vi "Excel_Update_Chart.vi"(0 "Excel._Worksheet":refnum<k7>, 1 "chart data":dbl[][](array[numeric]) format="%0.2f", 5 "Shapes":refnum<k7>, 9 "Chart index":u16, 11 "error in (no error)":errorcluster, 12 "column header":string[](array[string]), 13 "row header":string[](array[string])) -> (15 "error out":errorcluster)   [LabVIEW 2020, in "NI_ReportGenerationToolkit.lvlib"]
uses:
  <vilib>/addons/_office/NI_ReportGenerationToolkit.lvlib
panel:
  in  "MS Graph":refnum<k7>
  in  "Excel._OLEObject":refnum<k7>
  in  "Graph.Chart":refnum<k7>
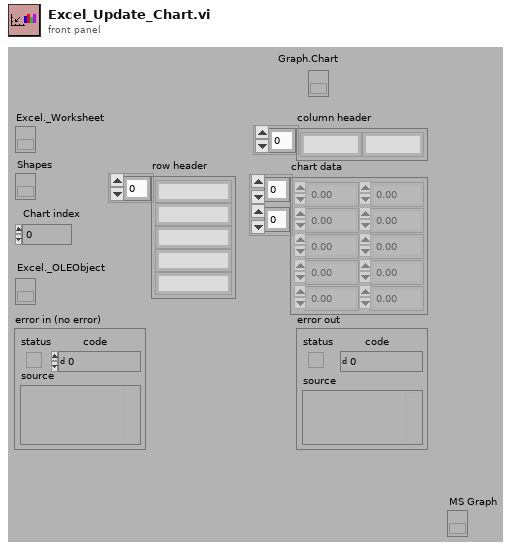
[diagram p1: front panel]
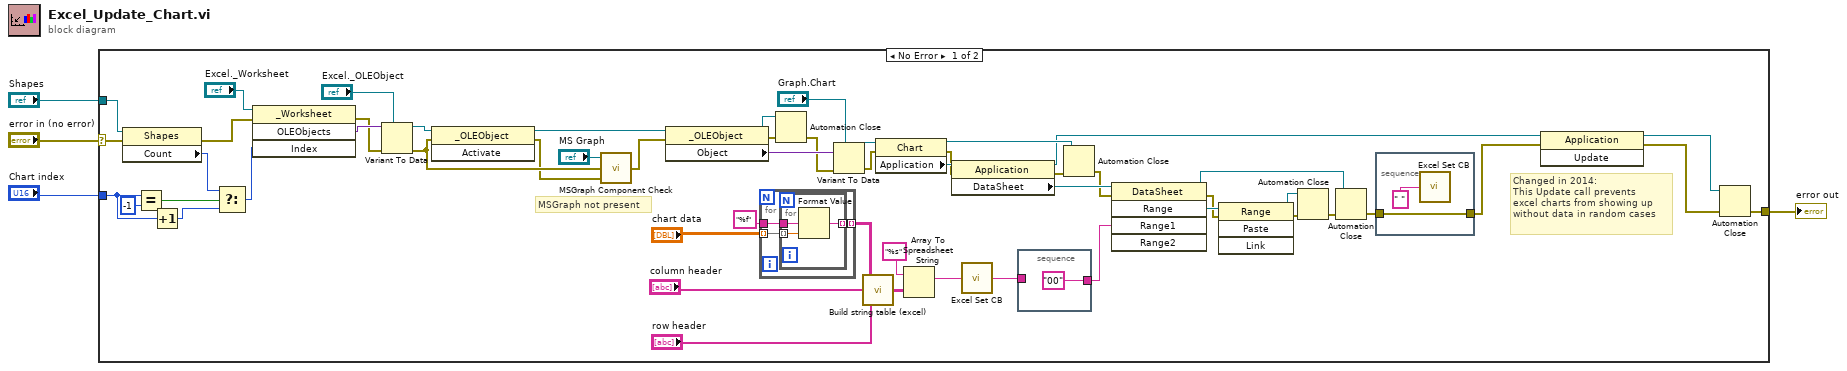
[diagram p0: block diagram]
diagram:
  n1 = case shown="No Error" "error in (no error)" {
    selector: "error in (no error)" -> [w9 w68]
    tunnel: "Chart index" -> [w46 _]
    tunnel: [w19 w68] -> w3
    tunnel: "Shapes" -> [w17 _]
    frame No Error {
      # "Changed in 2014:\nThis Update call prevents\nexcel charts from showing up \nwithout data in random cases"
      # "MSGraph not present"
      n2 = property class="Shapes"(reference=w17, error in=w9) -> (error out=w49:errorcluster, "Count"=w48:i32)  [unwired: 1 out]
      n3 = Equal?(x=w46, y=i16 -1) -> (x = y?=w57:bool)
      n4 = Increment(x=w46) -> (x+1=w55:u16)
      n5 = Select(t=w48, s=w57, f=w55) -> (s? t:f=w47:i32)
      n6 = invoke class="_Worksheet" method="OLEObjects"(reference="Excel._Worksheet", error in=w49, "Index"=w47) -> (error out=w52:errorcluster, "OLEObjects"=w53:variant)  [unwired: 1 in, 2 out]
      n7 = Variant To Data(error in=w52, type="Excel._OLEObject", Variant=w53) -> (data=w25:refnum<k7>, error out=w12:errorcluster)
      n8 = invoke class="_OLEObject" method="Activate"(reference=w25, error in=w12) -> (reference out=w24:refnum<k7>, error out=w11:errorcluster)  [unwired: 1 in, 1 out]
      n9 = call <vilib>:"MSGraph Component Check.vi"("error 2"=w11, "error 1"=w12, "MS Graph"="MS Graph") -> ("error out"=w10:errorcluster)
      n10 = property class="_OLEObject"(reference=w24, error in=w10) -> (reference out=w50:refnum<k7>, error out=w51:errorcluster, "Object"=w45:variant)
      n11 = for {
        tunnel: "chart data" -> [w64] mode=indexing
        tunnel: "%f" -> [w63]
        tunnel: [w62] -> w42 mode=indexing
        n12 = for {
          tunnel: w64 -> [w67] mode=indexing
          tunnel: w63 -> [w66]
          tunnel: [w65] -> w62 mode=indexing
          n13 = Format Value(format string=w66, value (0)=w67) -> (output string=w65:string)  [unwired: 1 out]
        }
      }
      n14 = Automation Close(3:w51, 5:w50) -> (0:w44:errorcluster)
      n15 = Variant To Data(error in=w44, type="Graph.Chart", Variant=w45) -> (data=w16:refnum<k7>, error out=w43:errorcluster)
      n16 = call <vilib>:"Build string table (excel).vi"("row headers"="row header", "column headers"="column header", "text data"=w42) -> ("output table"=w40:string[][])
      n17 = property class="Chart"(reference=w16, error in=w43) -> (reference out=w28:refnum<k7>, error out=w27:errorcluster, "Application"=w29:refnum<k7>)
      n18 = Array To Spreadsheet String(array=w40, 3:"%s" ("format string")) -> (spreadsheet string=w15:string)  [unwired: 1 out]
      n19 = property class="Application"(reference=w29, error in=w27) -> (reference out=w8:refnum<k7>, error out=w20:errorcluster, "DataSheet"=w32:refnum<k7>)
      n20 = call <vilib>:"Excel Set CB.vi"("String"=w15) -> ("String 2"=w14:string)
      n21 = stacked-sequence {
        tunnel: ["00"] -> w22
        tunnel: w14 -> [_]
        frame #0 {
        }
      }
      n22 = Automation Close(3:w20, 5:w28) -> (0:w31:errorcluster)
      n23 = invoke class="DataSheet" method="Range"(reference=w32, error in=w31, "Range1"=w22) -> (reference out=w34:refnum<k7>, error out=w33:errorcluster, "Range"=w35:refnum<k7>)  [unwired: 2 in, 2 out]
      n24 = invoke class="Range" method="Paste"(reference=w35, error in=w33) -> (reference out=w37:refnum<k7>, error out=w38:errorcluster)  [unwired: 2 in, 2 out]
      n25 = Automation Close(3:w38, 5:w37) -> (0:w36:errorcluster)
      n26 = Automation Close(3:w36, 5:w34) -> (0:w30:errorcluster)
      n27 = stacked-sequence {
        tunnel: w30 -> [w61]
        tunnel: [w61] -> w6
        frame #0 {
          n28 = call <vilib>:"Excel Set CB.vi"("String"=" ") -> ()  [unwired: 1 out]
        }
      }
      n29 = invoke class="Application" method="Update"(reference=w8, error in=w6) -> (reference out=w7:refnum<k7>, error out=w5:errorcluster)  [unwired: 1 in, 1 out]
      n30 = Automation Close(3:w5, 5:w7) -> (0:w19:errorcluster)
    }
    frame Error {
    }
  }
  "error out" <- w3
